vi "rad_Check Bitfile for AutoRun.vi"(8 "error in (no error)":errorcluster, 11 "path to XML document":path caption="path to bitfile") -> (0 "error out":errorcluster, 2 "AutoRun Text":string, 3 "AutoRun?":bool)   [LabVIEW 2014]
uses:
  <vilib>/xml/NI_XML.lvlib
  <vilib>/xml/Load XML File.vi
  <vilib>/xml/Close Reference(Node).vi
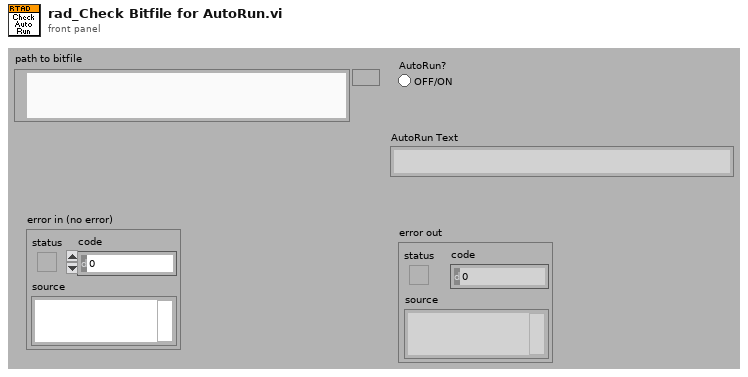
[diagram p1: front panel]
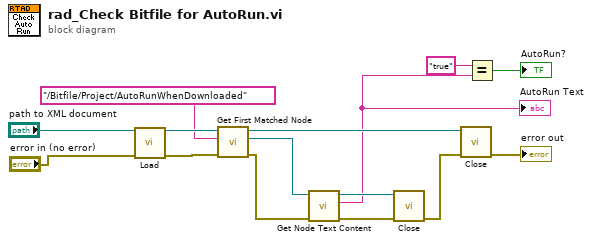
[diagram p0: block diagram]
diagram:
  n1 = call-poly <vilib>:"Load.vi"("path to XML document"="path to XML document", "error in (no error)"="error in (no error)") -> ("DOM document out"=w15:refnum<k20>, "error out"=w14:errorcluster)  [unwired: 11 in, 1 out]
  n2 = call <vilib>:"Get First Matched Node.vi"("error in (no error)"=w14, "XPath expression"="/Bitfile/Project/AutoRunWhenDownloaded", "node in"=w15) -> ("error out"=w10:errorcluster, "node result"=w11:refnum<k20>, "node out"=w6:refnum<k20>)  [unwired: 6 in]
  n3 = call <vilib>:"Get Node Text Content.vi"("error in (no error)"=w10, "node in"=w11) -> ("error out"=w9:errorcluster, "node text"=w4:string, "node out"=w8:refnum<k20>)  [unwired: 7 in]
  "AutoRun Text" <- w4
  n4 = call-poly <vilib>:"Close.vi"("error in (no error)"=w9, "node"=w8) -> ("error out"=w7:errorcluster)  [unwired: 7 in]
  n5 = call-poly <vilib>:"Close.vi"("error in (no error)"=w7, "node"=w6) -> ("error out"=→"error out":errorcluster)  [unwired: 7 in]
  n6 = Equal?(x="true", y=w4) -> (x = y?=→"AutoRun?":bool)
